vi "Big_LED_control.vi"() -> ()   [LabVIEW 2018]
uses:
  <instrlib>/niDCPower/nidcpower.llb/niDCPower Source Mode.ctl
  <instrlib>/niDCPower/nidcpower.llb/niDCPower Output Function.ctl
  AT lib/AmateurStepperMotor.dll
  <instrlib>/niDMM/nidmm.llb/niDMM Function.ctl
  <instrlib>/niDMM/nidmm.llb/niDMM Resolution in Digits.ctl
  <vilib>/Instr/_visa.llb/VISA Configure Serial Port (Instr).vi
  <instrlib>/niDMM/nidmm.llb/niDMM Configure Measurement Digits.vi
panel:
  out "Voltage Char 2":dbl(graph)=0.2558511793613434
  in  "I (np)":bool
  in  "Tab Control 2":enum32{"Шаговик и офир", "Служебная область"}(tab)
  in  "milliseconds to wait":u32=1000
  in  "Go To":dbl
  out "Ophir 1 Char":dbl(graph)=0.02
  in  "DecelerationTime, s":dbl=0.3
  in  "AccelerationTime, s":dbl=0.3
  in  "HoldOn":bool
  in  "Ophir 1 units":string(combo)="1000" caption="Units"
  out "Ophir 1 Over Range":bool caption="Over Range"
  out "Ophir 1 Optical Power":dbl=0.02 caption="Power" format="%#_4g"
  out "Ophir 1 MAX":dbl=0.02 caption="MAX" format="%#_5g"
  in  "Ophir 1 Clear":bool caption="Clear"
  in  "StepMultiplicationFactor":dbl=50.0
  in  "StepDivisor":i32(ring)=8 items=["D1"=1, "D2"=2, "D4"=4, "D8"=8, "D16"=16, "D32"=32]
  in  "Speed":dbl=250.0
  in  "Погнали!":bool
  in  "Стоп GoTo":bool
  out "Готово":bool
  out "Position":dbl=9.995
  in  "Ophir 1 Info":u16(ring)=1 caption="Info" items=["Device : ; s/n:", "Head : ; s/n:"]
  in  "new pos":dbl
  in  "set pos":bool
  out "Device Response":string="*\n"
  in  "Ophir 1 usb channel":i16 caption="usb channel"
  out "Ophir 1 dup Visa Session":refnum<visa-resource-name>="USB0::0x0BD3::0x0777::NI-VISA-60003::RAW" caption="dup Visa Session"
  in  "Ophir 1 Baud Rate (3:9600)":i16(ring)=3 caption="Baud Rate (3:9600)" items=["300", "1200", "4800", "9600", "19200", "38400"]
  out "Ophir 1 Real Optical Power":dbl=2e-05 format="%.6e"
  in  "Ophir 1 GPIB Address (10)":string="10" caption="GPIB Address (10)"
  in  "Ophir 1 Port Number (default 2)":i16=1 caption="Port Number (default 2)" min=0 max=20
  in  "Ophir 1 Select Communication Protocol":u16(ring) caption="Select Communication Protocol" items=["USB", "RS232", "GPIB"]
  out "Ophir 1 error out":errorcluster caption="error out"
  in  "Ophir 1 error in (no error)":errorcluster caption="error in (no error)"
  in  "Ophir 1 Wait":u32=100 caption="Wait"
  out "IsOpen":bool
  out "Ophir 1 Initialization":bool=TRUE caption="Initialization"
  in  "Tab Control":T1(tab)
  in  "шаговик":refnum<visa-resource-name>="COM8"
  in  "POWER":bool
  in  "Стоп":bool
  in  "Resource Name":refnum<k15>="PXI1Slot2" caption="Источник питания"
  in  "Амперметр":refnum<k15>="PXI1Slot4" caption="NI DMM 1"
  in  "V_MB, V":dbl=6.0 caption="voltage level" min=0.0 max=6.0 format="%_6p"
  in  "curlim_V_MB, A":dbl=0.3 caption="current limit" format="%_6p"
  out "chart_0":dbl(graph)=-0.00013853853853977013 caption="Waveform Chart 5"
  in  "voltlim_I_LED, V":dbl=2.1 caption="current limit" min=0.01 format="%_6p"
  in  "I_LED, A":dbl=0.010000000000000004 caption="voltage level" format="%_6p"
  out "chart_1":dbl(graph)=-0.0002744397184121777 caption="Waveform Chart 5"
  out "Current Char":dbl(graph)=0.0055655837059021
  in  "Arduino":refnum<visa-resource-name>="COM16"
  in  "Сегменты":bool[](array[boolean])=[FALSE, FALSE, FALSE, FALSE, FALSE, FALSE, FALSE, FALSE, FALSE, FALSE, FALSE, FALSE, FALSE, FALSE, FALSE, FALSE, FALSE, FALSE]
  in  "Вольтметр":refnum<k15>="PXI1Slot5" caption="NI DMM 1"
  out "Voltage Char":dbl(graph)=0.2558511793613434
  in  "wave_lenght":string="600"
  in  "Промер":bool caption="Промер сегмента"
  in  "NI DMM 1 Voltage Range 4":string(combo)="-1" caption="Range"
  in  "NI DMM 1 units 4":string(combo)="1" caption="Units"
  out "Voltage":dbl=0.2558511793613434 format="%_6g"
  in  "NI DMM 1 Current Range 3":string(combo)="1" caption="Range"
  in  "NI DMM 1 units 3":string(combo)="1000" caption="Units"
  out "Current":dbl format="%_6g"
  out "voltmes_V_MB, V":dbl=-0.00013853853853977013 caption="measurement" format="%_6g"
  out "curmes_V_MB, A":dbl caption="measurement" format="%_6g"
  out "curmes_I_LED, A":dbl=9.117163901385412e-07 caption="measurement" format="%_6g"
  out "voltmes_I_LED, V":dbl caption="measurement" format="%_6g"
  out "Разряд":dbl
  out "+/-":bool
  out "Power off":bool
  in  "Command":string="Cathode"
  in  "Записать":bool
  out "measure output \nfile refnum":refnum<file>
  out "Voltage, V":dbl=0.2558511793613434 caption="Measurement" format="%.5f"
  out "Current, A":dbl=5.5655837059021e-06 caption="Measurement" format="%.5f"
  out "Тип индикатора":string="Cathode"
  out "chart_2":dbl(graph)=0.0007584113885058215
  in  "V_RES, V":dbl caption="voltage level" format="%_6p"
  out "curmes_V_RES, A":dbl caption="measurement" format="%_6g"
  in  "curlim_V_RES, A":dbl=0.1 caption="current limit" min=0.01 format="%_6p"
  in  "measure path":path=path "C:/Users/user/Desktop/МСП/LabVIEW/LED_CONTROL_big_LED_ophir_24.12.24_1/Logs"
  out "Enum":enum16{"Exit", "4", "Промер", "2", "1"}(ring)
  out "№ об-ца":dbl
  out "Темп-ра":dbl
  out "Сегмент":string="n"
  out "voltmes_V_RES, V":dbl=0.0007584113885058215 caption="measurement" format="%_6g"
  in  "current level range":dbl=0.001 format="%#.6p"
  in  "1 - до 10 мА\n0 - от  30 мА":bool
  in  "II (Lm)":bool
  in  "III (jk)":bool
  in  "IV (gh)":bool
  in  "I - IV":bool
  # "Шаговик"
  # "Офир"
  # "(в мм)"
  # "Шаговик"
  # "Офир"
  # "position - это значение абсолютное"
  # "*если нужен ток меньше 10мА -> служебная область"
  # "j"
  # "c"
  # "d"
  # "e"
  # "g"
  # "h"
  # "a"
  # "b"
  # "f"
  # "k"
  # "L"
  # "m"
  # "n"
  # "p"
  # "dp"
  # "all"
  # "V_MB 5 В\nогрничение 300 м\n\nV_LED 2,1 В\nограничение 200 м"
  # "единицы мА\nrange 1 А"
  # "1. каждый сегмент включаем по отдельности, резистором постраиваем ток до 10 мА\n2. напряжение V_LED при этом не меняется\n3. в такоом положении промеряем сегменты по отдельности\n4. для промера всего индикатора сразу подстраиваем напряжение при неизменном положении резисторов\n5. ток всех индикаторов = ток одного сегмента (10 мА) * число сегментов (15)\n6. добиваемся этого увеличением V_LED"
  # "единицы В\nrange AUTO"
  # "регклировка суммарного тока через индикатор"
  # "24.063\n\n     I          U\n20 мА  1.3 В\n20 мА  1.4 В\n 7 мА   1.15 В"
  # "24.064\n\n     I          U\n10 мА  2 В\n10 мА  2.15 В\n 7 мА   1.9 В"
  # "автоматизировать подбор напряжения по известному максимальному напряжению и току. ОС по току сегмента"
  # "Р1:  +25°C\nР2:  - 60°C\nР3:  +85°C"
  # "регулировать ток в зависимости от температуры.\nс ростом температуры растет ток.\nпид-регулятор??"
  # "0. ввести номер образца\n1. включить нужный сегмент\n2. ввести его в поле справа\n3. вести температуру в поле слева\n4. нажать кнопку \"промер сегмента\""
  # "\"опрашивать кнопки не чаще, чем раз в секунду. сейчас кликать можно чаще, они загорятся, но ничего не произойдет\""
  # "24.067"
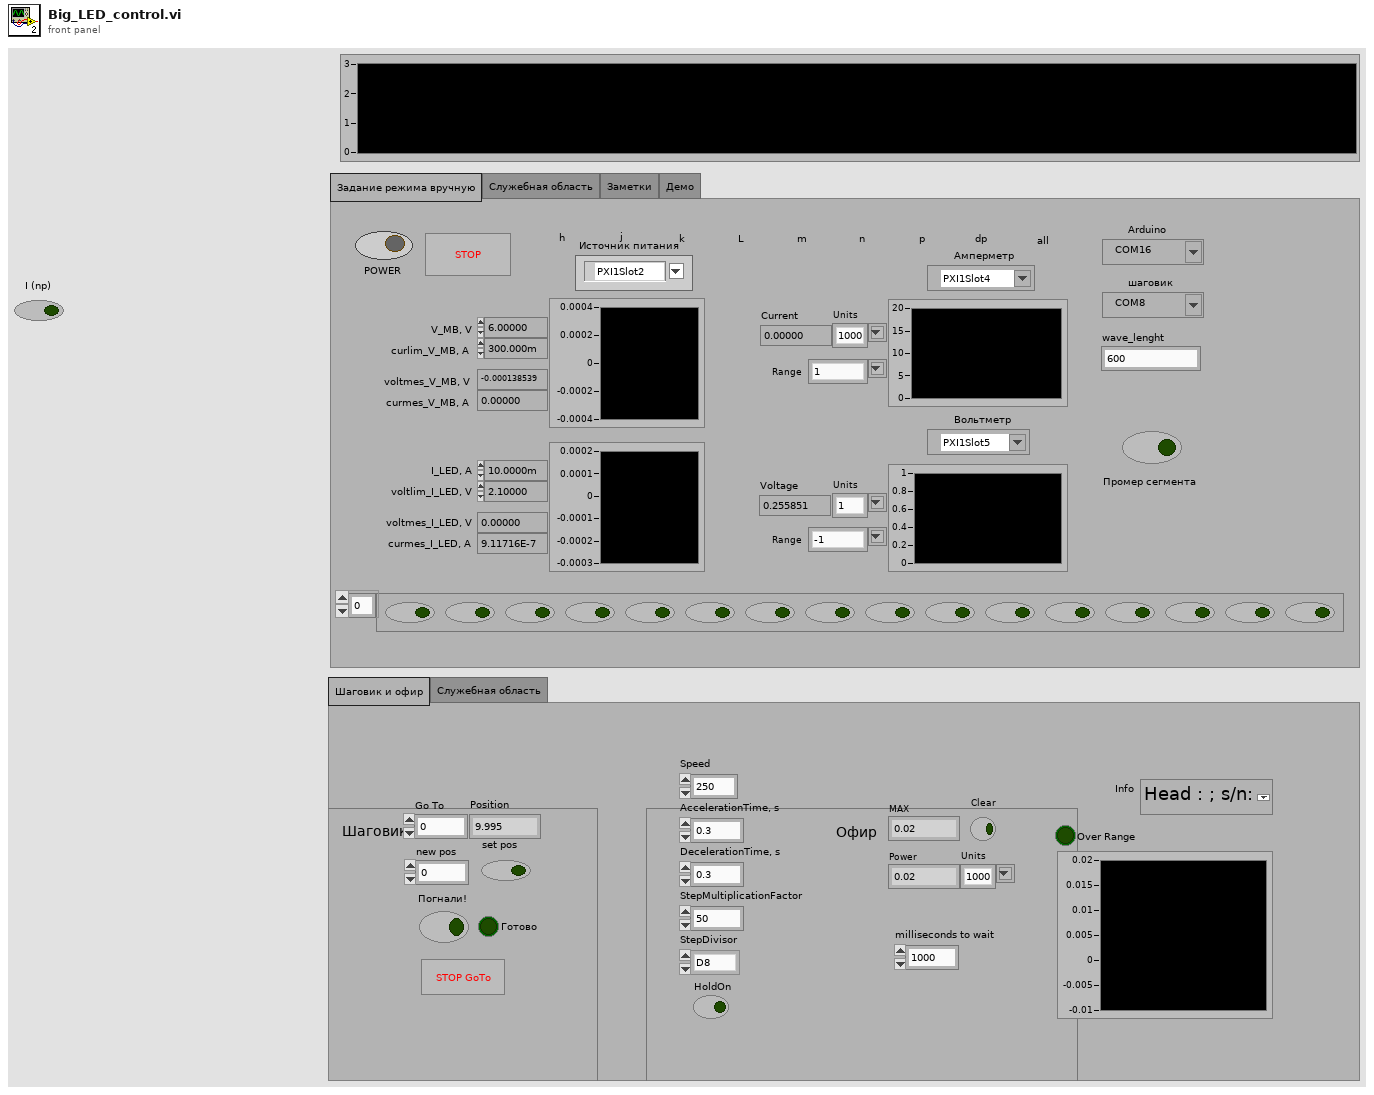
[diagram p1: front panel]
types:
  T1 = enum32{"Задание режима вручную", "Служебная область", "Заметки", "Демо"}
  T2 = enum16{"open", "replace", "create", "open or create", "replace or create", "replace or create with confirmation"}
  T3 = typedef "niDCPower Output Function.ctl" = i32
  T4 = typedef "niDCPower Source Mode.ctl" = i32
  T5 = typedef "niDMM Function.ctl" = enum16{"DC Volts", "AC Volts", "DC Current", "AC Current", "2-wire Resistance", "4-wire Resistance", "Diode", "Frequency", "Period", "AC Volts DC Coupled", "Capacitance", "Inductance", "Temperature"}
  T6 = typedef "niDMM Resolution in Digits.ctl" = dbl
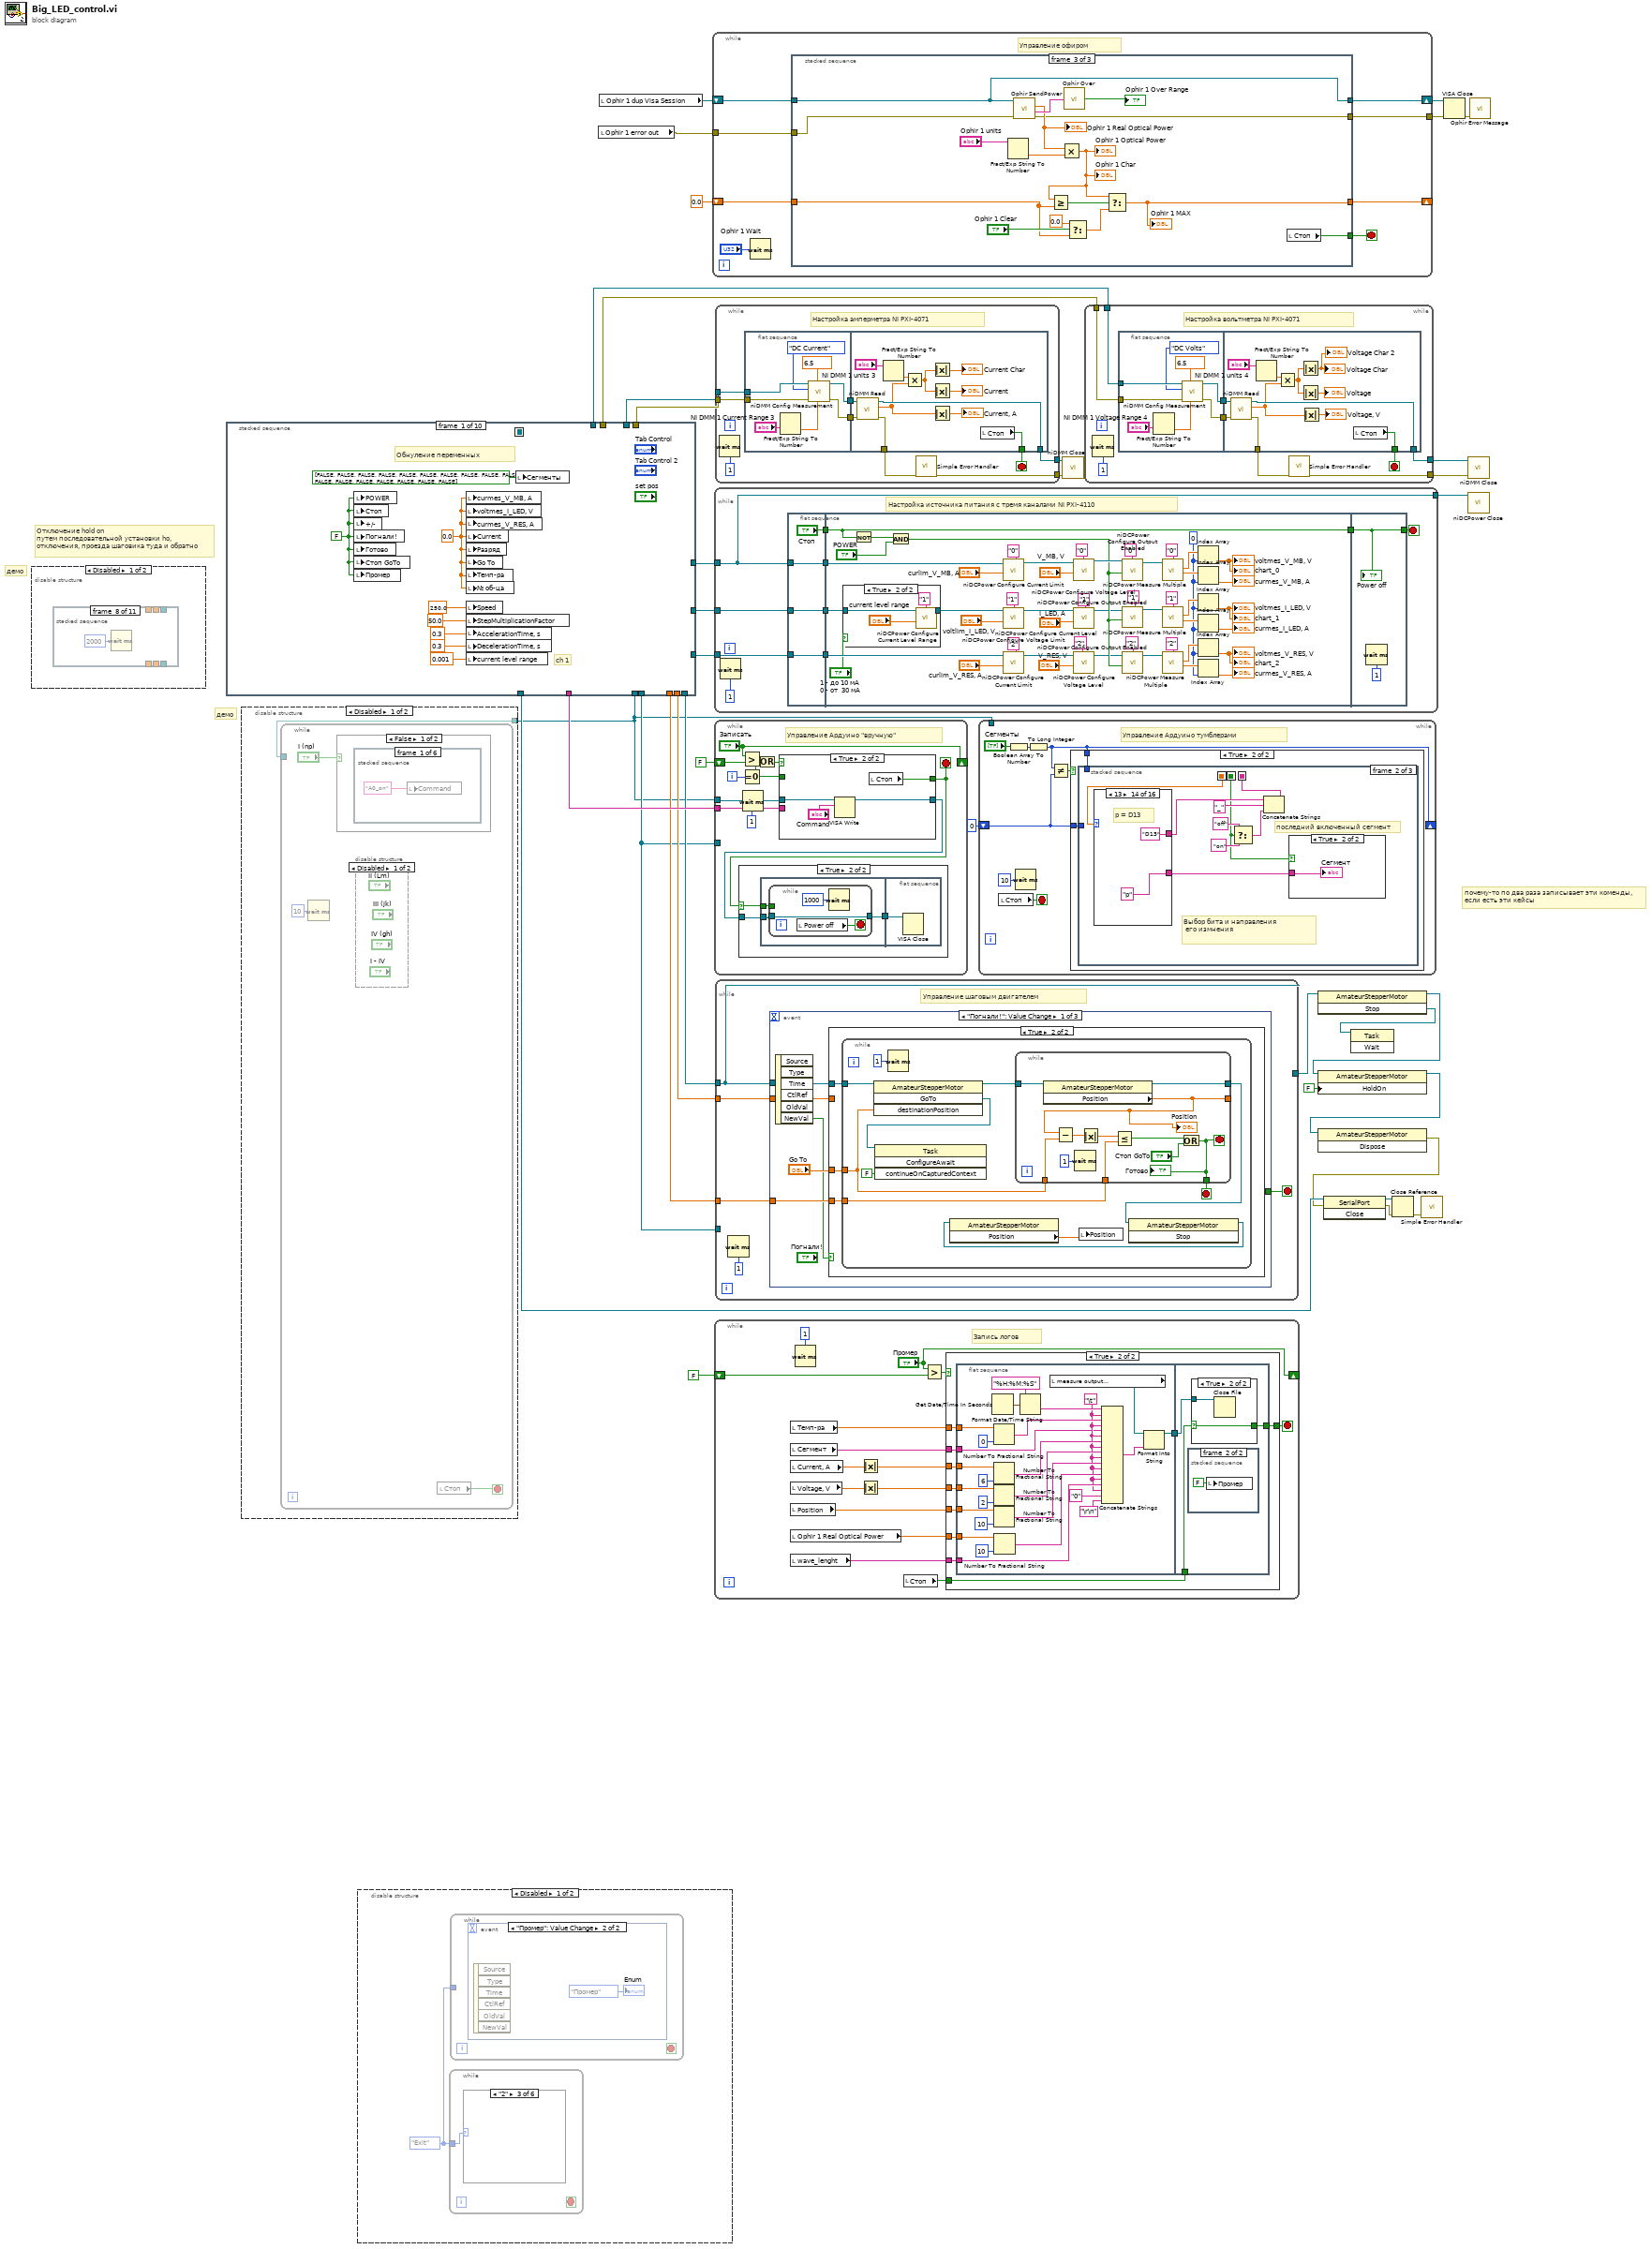
[diagram p0: block diagram]
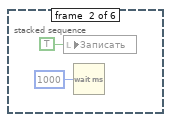
[diagram p3: hidden frame]
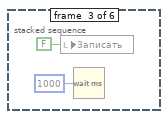
[diagram p4: hidden frame]
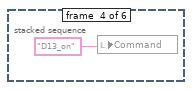
[diagram p5: hidden frame]
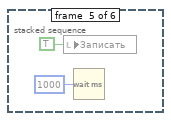
[diagram p6: hidden frame]
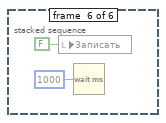
[diagram p7: hidden frame]
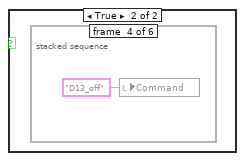
[diagram p8: hidden frame]
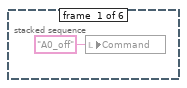
[diagram p9: hidden frame]
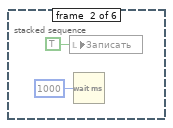
[diagram p10: hidden frame]
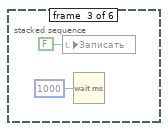
[diagram p11: hidden frame]
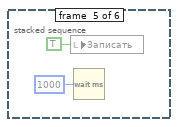
[diagram p12: hidden frame]
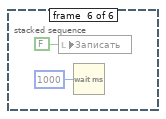
[diagram p13: hidden frame]
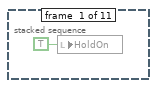
[diagram p15: hidden frame]
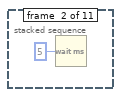
[diagram p16: hidden frame]
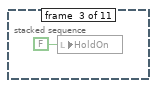
[diagram p17: hidden frame]
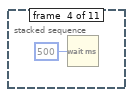
[diagram p18: hidden frame]
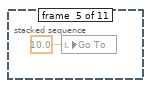
[diagram p19: hidden frame]
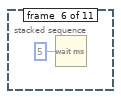
[diagram p20: hidden frame]
diagram:
  # "демо"
  # "демо"
  # "почему-то по два раза записывает эти коменды,\nесли есть эти кейсы"
  # "Отключение hold on\nпутем последовательной установки ho, \nотключения, проезда шаговика туда и обратно"
  n1 = disable-structure shown="Disabled" {
    frame Disabled {
      n2 = stacked-sequence {
        tunnel: _ -> [_ _ _ _ _ _ _ _ _ _ w50]
        tunnel: [_ _ _ _ _ _ _ _ _ _ w50] -> _
        tunnel: _ -> [_ _ _ _ _ _ _ _ _ _ w49]
        tunnel: [_ _ _ _ _ _ _ _ _ _ w49] -> _
        tunnel: [_ _ _ _ _ _ _ _ _ _ w48] -> _
        tunnel: _ -> [_ _ _ _ _ _ _ _ _ _ w48]
        frame #0 {
          n3 = local write "HoldOn"(TRUE ("HoldOn")) -> ()
        }
        frame #1 {
          n4 = Wait (ms)(milliseconds to wait=u32 5) -> ()  [unwired: 1 out]
        }
        frame #2 {
          n5 = local write "HoldOn"(FALSE ("HoldOn")) -> ()
        }
        frame #3 {
          n6 = Wait (ms)(milliseconds to wait=u32 500) -> ()  [unwired: 1 out]
        }
        frame #4 {
          n7 = local write "Go To"(10.0 ("Go To")) -> ()
        }
        frame #5 {
          n8 = Wait (ms)(milliseconds to wait=u32 5) -> ()  [unwired: 1 out]
        }
        frame #6 {
          n9 = local write "Погнали!"(TRUE ("Погнали!")) -> ()
        }
        frame #7 {
          n10 = Wait (ms)(milliseconds to wait=u32 2000) -> ()  [unwired: 1 out]
        }
        frame #8 {
          n11 = local write "Go To"(0.0 ("Go To")) -> ()
        }
        frame #9 {
          n12 = Wait (ms)(milliseconds to wait=u32 5) -> ()  [unwired: 1 out]
        }
        frame #10 {
          n13 = local write "Погнали!"(TRUE ("Погнали!")) -> ()
        }
      }
    }
    frame Enabled {
    }
  }
  n14 = stacked-sequence {
    seq-local: [_ _ _ _ _ _ w113 _ _ _] -> [_ _ _ _ _ _ _ w138 _ _]
    tunnel: [_ _ _ w68 _ _ _ _ _ _] -> w26
    tunnel: [_ w62 _ _ _ _ _ _ _ _] -> w37
    tunnel: [_ w61 _ _ _ _ _ _ _ _] -> w36
    tunnel: [_ _ _ _ w88 _ _ _ _ _] -> w1
    tunnel: [_ _ _ _ _ _ _ _ w144 _] -> w33
    tunnel: [_ _ w65 _ _ _ _ _ _ _] -> w32
    tunnel: [_ _ w64 _ _ _ _ _ _ _] -> w31
    tunnel: [_ _ _ _ _ _ _ w141 _ _] -> w3
    tunnel: [_ _ _ _ _ _ _ w139 _ _] -> w4
    tunnel: [_ _ _ _ _ _ _ w140 _ _] -> w5
    tunnel: [_ _ _ _ _ _ w115 _ _ _] -> w20
    tunnel: [_ _ _ w67 _ _ _ _ _ _] -> w8
    tunnel: [_ _ _ w66 _ _ _ _ _ _] -> w6
    tunnel: [_ _ _ _ _ _ _ _ _ w145] -> w2
    frame #0 {
      w52 = 0.0 ("currentmes_2")
      w53 = FALSE ("Стоп")
      # "ch 1"
      # "Обнуление переменных"
      n15 = local write "POWER"(w53) -> ()
      n16 = local write "Стоп"(w53) -> ()
      n17 = local write "+/-"(w53) -> ()
      n18 = local write "Погнали!"(w53) -> ()
      n19 = local write "Готово"(w53) -> ()
      n20 = local write "Стоп GoTo"(w53) -> ()
      n21 = local write "Промер"(w53) -> ()
      n22 = local write "curmes_V_MB, A"(w52) -> ()
      n23 = local write "voltmes_I_LED, V"(w52) -> ()
      n24 = local write "curmes_V_RES, A"(w52) -> ()
      n25 = local write "Current"(w52) -> ()
      n26 = local write "Разряд"(w52) -> ()
      n27 = local write "Go To"(w52) -> ()
      n28 = local write "Темп-ра"(w52) -> ()
      n29 = local write "№ об-ца"(w52) -> ()
      n30 = local write "Speed"(250.0 ("Speed")) -> ()
      n31 = local write "StepMultiplicationFactor"(50.0 ("StepMultiplicationFactor")) -> ()
      n32 = local write "AccelerationTime, s"(0.3 ("AccelerationTime, s")) -> ()
      n33 = local write "DecelerationTime, s"(0.3 ("DecelerationTime, s")) -> ()
      n34 = local write "current level range"(0.001 ("current level range")) -> ()
      n35 = local write "Сегменты"(bool[] [FALSE, FALSE, FALSE, FALSE, FALSE, FALSE, FALSE, FALSE, FALSE, FALSE, FALSE, FALSE, FALSE, FALSE, FALSE, FALSE, FALSE, FALSE] ("Сегменты")) -> ()
    }
    frame #1 {
      # "Инициализация амперметра"
      n36 = call <instrlib>:"niDMM Initialize.vi"("Instrument Descriptor"="Амперметр") -> ("error out"=w62:errorcluster, "instrument handle out"=w61:refnum<k15>)  [unwired: 9 in]
    }
    frame #2 {
      # "Инициализация вольтметра"
      n37 = call <instrlib>:"niDMM Initialize.vi"("Instrument Descriptor"="Вольтметр") -> ("error out"=w64:errorcluster, "instrument handle out"=w65:refnum<k15>)  [unwired: 9 in]
    }
    frame #3 {
      w73 = T3 1006 items=["DC Voltage"=1006, "DC Current"=1007, "Pulse Voltage"=1049, "Pulse Current"=1050] ("output function")
      w77 = T3 1007 items=["DC Voltage"=1006, "DC Current"=1007, "Pulse Voltage"=1049, "Pulse Current"=1050] ("output function")
      w78 = T3 1006 items=["DC Voltage"=1006, "DC Current"=1007, "Pulse Voltage"=1049, "Pulse Current"=1050] ("output function")
      w81 = T4 1020 items=["Single Point"=1020, "Sequence"=1021] ("source mode")
      # "Инициализация источника питания"
      n38 = call <instrlib>:"niDCPower Initialize.vi"("resource name"="Resource Name") -> ("instrument handle out"=w82:refnum<k15>)  [unwired: 3 in, 7 out]
      n39 = call <instrlib>:"niDCPower Configure Source Mode.vi"("source mode"=w81, "instrument handle"=w82) -> ("instrument handle out"=w72:refnum<k15>)  [unwired: 1 in, 8 out]
      n40 = call <instrlib>:"niDCPower Configure Output Function.vi"("output function"=w77, "channel name"="1", "instrument handle"=w72) -> ("instrument handle out"=w79:refnum<k15>)  [unwired: 7 in, 1 out]
      n41 = call <instrlib>:"niDCPower Configure Output Function.vi"("output function"=w73, "channel name"="2", "instrument handle"=w72) -> ("instrument handle out"=w74:refnum<k15>)  [unwired: 7 in, 1 out]
      n42 = call <instrlib>:"niDCPower Configure Output Function.vi"("output function"=w78, "channel name"="0", "instrument handle"=w72) -> ("instrument handle out"=w80:refnum<k15>)  [unwired: 7 in, 1 out]
      n43 = call <instrlib>:"niDCPower Configure Voltage Level.vi"("voltage level"=0.0, "channel name"="2", "instrument handle"=w74) -> ("instrument handle out"=w66:refnum<k15>)  [unwired: 7 in, 1 out]
      n44 = call <instrlib>:"niDCPower Configure Voltage Level.vi"("voltage level"=0.0, "channel name"="0", "instrument handle"=w80) -> ("instrument handle out"=w68:refnum<k15>)  [unwired: 7 in, 1 out]
      n45 = call <instrlib>:"niDCPower Configure Current Level.vi"("current level"=0.01, "channel name"="1", "instrument handle"=w79) -> ("instrument handle out"=w67:refnum<k15>)  [unwired: 7 in, 1 out]
    }
    frame #4 {
      # "Инициализация Ардуино"
      n46 = call-poly "VISA Configure Serial Port"("VISA resource name"="Arduino", "baud rate (9600)"=u32 9600) -> ("VISA resource name out"=w88:refnum<visa-resource-name>)  [unwired: 12 in, 1 out]
    }
    frame #5 {
      # "Инициализация офира"
      n47 = call "Ophir InitCom.vi"("GPIB Address (default 10)"="Ophir 1 GPIB Address (10)", "Communication (default USB 0)"="Ophir 1 Select Communication Protocol", "USB Channel number (default 0)"="Ophir 1 usb channel", "Port Number (default 2)"="Ophir 1 Port Number (default 2)", "error in (no error)"="Ophir 1 error in (no error)", "Baud Rate (3:9600)"="Ophir 1 Baud Rate (3:9600)") -> ("dup Visa Session"=w97:refnum<visa-resource-name>, "error out"=w96:errorcluster)  [unwired: 1 out]
      n48 = call "Ophir InstrInfo.vi"("Visa Session"=w97, "error in (no error)"=w96) -> ("dup Visa Session"=w109:refnum<visa-resource-name>, "Instrument Info"=w91:string, "error out"=w107:errorcluster)
      n49 = call "Ophir HeadInfo.vi"("Visa Session"=w109, "error in (no error)"=w107) -> ("error out"=w106:errorcluster, "dup Visa Session"=w108:refnum<visa-resource-name>, "Head Info"=w105:string)  [unwired: 6 out]
      n50 = call "Ophir InfoStrings.vi"("error in (no error)"=w106, "Head Info"=w105, "Instrument Info"=w91) -> ("error out"=w104:errorcluster, "Strings Array"=w103:string[])
      n51 = property on="Ophir 1 Info" class="Ring (strict)"("Strings []"=w103) -> ()  [unwired: 2 in, 2 out]
      n52 = call "Ophir ConfigDevice.vi"("Visa Session"=w108, "Measure Choice (0:Power)"=u16 0, "error in (no error)"=w104) -> ("dup Visa Session"=→"Ophir 1 dup Visa Session":refnum<visa-resource-name>, "OK ?"=→"Ophir 1 Initialization":bool, "error out"=→"Ophir 1 error out":errorcluster)  [unwired: 1 out]
    }
    frame #6 {
      w120 = 100 ("WriteTimeout")
      w124 = 1 items=["None", "One", "Two", "OnePointFive"] ("stopBits")
      w122 = 0 items=["None", "Odd", "Even", "Mark", "Space"] ("parity")
      # "убрали открытие порта. шаговик его и так сам откроет"
      # "Инициализация шаговика ч.1"
      n53 = constructor class="SerialPort"("portName"="шаговик", "baudRate"=57600, "parity"=w122, "dataBits"=8, "stopBits"=w124) -> (reference out=w119:refnum<k24>, error out=w118:errorcluster)  [unwired: 3 in, 6 out]
      n54 = property class="SerialPort"(reference=w119, error in=w118, "WriteTimeout"=w120, "ReadTimeout"=w120) -> (reference out=w115:refnum<k24>)  [unwired: 1 out]
      n55 = flat-sequence {
        tunnel: w115 -> [w131]
        tunnel: w114 -> [_]
        frame #0 {
          n56 = property class="SerialPort"(reference=w131) -> ("IsOpen"=→"IsOpen":bool)  [unwired: 1 in, 2 out]
        }
      }
      n57 = constructor class="AmateurStepperMotor"("serialPort"=w115) -> (reference out=w112:refnum<k24>, error out=w111:errorcluster)  [unwired: 3 in, 2 out]
      n58 = Not A Number/Path/Refnum?(number/path/refnum=w112) -> (NaN/Path/Refnum?=w116:bool)
      n59 = case shown="False" w116 {
        tunnel: w115 -> [_ w129]
        tunnel: [w125 w128] -> w114
        tunnel: [w126 w127] -> w113
        tunnel: w112 -> [w126 _]
        tunnel: w111 -> [w125 _]
        frame False {
        }
        frame True {
          n60 = constructor class="AmateurStepperMotor"("serialPort"=w129) -> (reference out=w127:refnum<k24>, error out=w128:errorcluster)  [unwired: 3 in, 2 out]
        }
      }
    }
    frame #7 {
      # "стоит допустить изменение\nтих параметров в цикле, а не только \nпри инициализации"
      # "это те самые 50 шагов за мм"
      # "Инициализация шаговика ч.2"
      n61 = property class="AmateurStepperMotor"(reference=w138, "Speed"="Speed", "StepDivisor"="StepDivisor", "StepMultiplicationFactor"="StepMultiplicationFactor", "AccelerationTime"="AccelerationTime, s", "DecelerationTime"="DecelerationTime, s", "HoldOn"="HoldOn") -> (reference out=w141:refnum<k24>, "Position"=w139:dbl, "PositioningPrecision"=w140:dbl)  [unwired: 1 in, 1 out]
    }
    frame #8 {
      # "Begin VI: ОК или ОА?"
      n62 = call "Begin.vi"() -> ("Темп-ра"=→"Темп-ра":dbl, "№ об-ца"=→"№ об-ца":dbl, "String"=w144:string)  [unwired: 6 in]
      "Тип индикатора" <- w144
      n63 = local write "Command"(w144) -> ()
    }
    frame #9 {
      w155 = "\t"
      # "Инициализация логов"
      n64 = local read "№ об-ца"() -> (w159:dbl)
      n65 = Number To Fractional String(number=w159, precision (6)=i16 0) -> (F-format string=w160:string)  [unwired: 2 in]
      n66 = Get Date/Time In Seconds() -> (seconds since 1Jan1904=w170:timestamp)
      n67 = Build Path(base path="measure path", name or relative path=w160) -> (appended path=w166:path)
      n68 = call <vilib>:"Check if File or Folder Exists.vi"("path"=w166) -> ("file or folder exists?"=w167:bool, "dup path"=w168:path)  [unwired: 8 in, 1 out]
      n69 = Format Date/Time String(time format string (%c)="MES %d. %m. %y %H.%M.%S", seconds (now)=w170) -> (date/time string=w171:string)  [unwired: 1 in]
      n70 = case shown="True" w167 {
        tunnel: w168 -> [w177 w178]
        tunnel: [w176 w178] -> w169
        frame False {
          n71 = Create Folder(path (use dialog)=w177) -> (created path=w176:path)  [unwired: 2 in, 2 out]
        }
        frame True {
        }
      }
      n72 = Concatenate Strings(w171, ".xls" ("string")) -> (w172:string)
      n73 = Build Path(base path=w169, name or relative path=w172) -> (appended path=w173:path)
      n74 = Open/Create/Replace File(file path (use dialog)=w173, operation (0:open)=T2."open or create", access (0:read/write)=enum16{"read/write", "read-only", "write-only"}."read/write") -> (refnum out=w174:refnum<file>)  [unwired: 3 in, 2 out]
      n75 = Set File Position(refnum=w174, from (0:start)=enum16{"start", "end", "current"}."end") -> (refnum out=w157:refnum<file>)  [unwired: 2 in, 1 out]
      n76 = Format Into String(initial string=w157, "Time" ("string"), w155, "Temperature, C" ("string"), w155, "Segment" ("string"), w155, "Current, mA" ("string"), w155, "Voltage, V" ("input 7"), w155, "Distance, m" ("string"), w155, "Power, W " ("string"), w155, "Wavelenght, nm" ("input 17"), w155, "Candlepower, kd" ("string"), "\r\n") -> (resulting string=w145:refnum<file>)  [unwired: 2 in, 1 out]
      "measure output \nfile refnum" <- w145
    }
  }
  n77 = disable-structure shown="Disabled" {
    disable-tunnel: w1 -> [w179 _]
    frame Disabled {
      n78 = while {
        tunnel: w179 -> [_]
        stop <- w181 stop-if-true
        n79 = Wait (ms)(milliseconds to wait=u32 10 ("millisecond timer value")) -> ()  [unwired: 1 out]
        n80 = case shown="False" "I (np)" {
          frame False {
            n81 = stacked-sequence {
              frame #0 {
                n82 = local write "Command"("A0_on" ("Command")) -> ()
              }
              frame #1 {
                n83 = local write "Записать"(TRUE ("Записать")) -> ()
                n84 = Wait (ms)(milliseconds to wait=u32 1000) -> ()  [unwired: 1 out]
              }
              frame #2 {
                n85 = local write "Записать"(FALSE ("Записать")) -> ()
                n86 = Wait (ms)(milliseconds to wait=u32 1000) -> ()  [unwired: 1 out]
              }
              frame #3 {
                n87 = local write "Command"("D13_on" ("Command")) -> ()
              }
              frame #4 {
                n88 = local write "Записать"(TRUE ("Записать")) -> ()
                n89 = Wait (ms)(milliseconds to wait=u32 1000) -> ()  [unwired: 1 out]
              }
              frame #5 {
                n90 = local write "Записать"(FALSE ("Записать")) -> ()
                n91 = Wait (ms)(milliseconds to wait=u32 1000) -> ()  [unwired: 1 out]
              }
            }
          }
          frame True {
            n92 = stacked-sequence {
              frame #0 {
                n93 = local write "Command"("A0_off" ("Command")) -> ()
              }
              frame #1 {
                n94 = local write "Записать"(TRUE ("Записать")) -> ()
                n95 = Wait (ms)(milliseconds to wait=u32 1000) -> ()  [unwired: 1 out]
              }
              frame #2 {
                n96 = local write "Записать"(FALSE ("Записать")) -> ()
                n97 = Wait (ms)(milliseconds to wait=u32 1000) -> ()  [unwired: 1 out]
              }
              frame #3 {
                n98 = local write "Command"("D13_off" ("Command")) -> ()
              }
              frame #4 {
                n99 = local write "Записать"(TRUE ("Записать")) -> ()
                n100 = Wait (ms)(milliseconds to wait=u32 1000) -> ()  [unwired: 1 out]
              }
              frame #5 {
                n101 = local write "Записать"(FALSE ("Записать")) -> ()
                n102 = Wait (ms)(milliseconds to wait=u32 1000) -> ()  [unwired: 1 out]
              }
            }
          }
        }
        n103 = disable-structure shown="Disabled" {
          frame Disabled {
          }
          frame Enabled {
          }
        }
        n104 = local read "Стоп"() -> (w181:bool)
      }
    }
    frame Enabled {
    }
  }
  n105 = disable-structure shown="Disabled" {
    frame Disabled {
      w203 = enum16{"Exit", "4", "Промер", "2", "1"}."Exit"
      n106 = while {
        tunnel: w203 -> [w204]
        stop <- _ stop-if-true
        n107 = case shown="\"2\"" w204 {
          frame "Exit", Default {
          }
          frame "4" {
          }
          frame "2" {
          }
          frame "2" {
          }
          frame "1" {
          }
          frame "Промер" {
          }
        }
      }
      n108 = while {
        tunnel: w203 -> [_]
        stop <- _ stop-if-true
        n109 = event shown="[1] \"Промер\": Value Change" {
          selector: _ -> [_ _]
          dyn-events: _ -> [_ _]
          timeout: _ -> [_ _]
          event Timeout {
            n110 = event-data() -> ()  [unwired: 1 in, 3 out]
          }
          event "Промер": Value Change {
            n111 = event-data() -> ()  [unwired: 1 in, 6 out]
            "Enum" <- enum16{"Exit", "4", "Промер", "2", "1"}."Промер" ("Enum")
          }
        }
      }
    }
    frame Enabled {
    }
  }
  n112 = local read "Ophir 1 error out"() -> (w24:errorcluster)
  n113 = local read "Ophir 1 dup Visa Session"() -> (w25:refnum<visa-resource-name>)
  n114 = while {
    tunnel: w24 -> [w212]
    shift-right: [w208] -> _
    shift-left: 0.0 ("t") -> [w211]
    shift-right: [w209] -> w18
    shift-left: w25 -> [w213]
    tunnel: [w207] -> w17
    stop <- w206 stop-if-true
    # "Управление офиром"
    n115 = Wait (ms)(milliseconds to wait="Ophir 1 Wait") -> ()  [unwired: 1 out]
    n116 = stacked-sequence {
      tunnel: w213 -> [w217 _ w220]
      tunnel: w212 -> [w216 _ w222]
      tunnel: w211 -> [_ _ w223]
      tunnel: [_ _ w220] -> w209
      tunnel: [_ _ w224] -> w208
      tunnel: [_ _ w221] -> w207
      tunnel: [_ _ w219] -> w206
      frame #0 {
        n117 = call "light_setWaveLenght.vi"("error in (no error)"=w216, "Visa Session"=w217, "wave_lenght"="wave_lenght") -> ("Device Response"=→"Device Response":string)  [unwired: 6 in, 2 out]
      }
      frame #1 {
        n118 = Wait (ms)(milliseconds to wait="milliseconds to wait") -> ()  [unwired: 1 out]
      }
      frame #2 {
        n119 = Fract/Exp String To Number(string="Ophir 1 units") -> (number=w227:dbl)  [unwired: 3 in, 1 out]
        n120 = call "Ophir SendPower.vi"("Visa Session"=w220, "error in (no error)"=w222) -> ("Value Number"=w226:dbl, "Value String"=w233:string, "error out"=w221:errorcluster)  [unwired: 1 out]
        "Ophir 1 Real Optical Power" <- w226
        n121 = Multiply(x=w226, y=w227) -> (x*y=w230:dbl)
        "Ophir 1 Char" <- w230
        "Ophir 1 Optical Power" <- w230
        n122 = Greater Or Equal?(x=w230, y=w223) -> (x >= y?=w231:bool)
        n123 = call "Ophir Over.vi"("Value String"=w233) -> ("Overrange"=→"Ophir 1 Over Range":bool)
        n124 = Select(t=0.0, s="Ophir 1 Clear", f=w223) -> (s? t:f=w229:dbl)
        n125 = Select(t=w230, s=w231, f=w229) -> (s? t:f=w224:dbl)
        "Ophir 1 MAX" <- w224
        n126 = local read "Стоп"() -> (w219:bool)
      }
    }
  }
  n127 = while {
    tunnel: w26 -> [w241]
    tunnel: [w241] -> w34
    tunnel: w8 -> [w238]
    tunnel: w6 -> [w235]
    stop <- w237 stop-if-true
    # "Настройка источника питания с тремя каналами NI PXI-4110"
    n128 = Wait (ms)(milliseconds to wait=u32 1) -> ()  [unwired: 1 out]
    n129 = flat-sequence {
      tunnel: w241 -> [w248]
      tunnel: [w248] -> w243
      tunnel: ["Стоп"] -> w242
      tunnel: [w246] -> w239
      tunnel: w238 -> [w246]
      tunnel: [w245] -> w236
      tunnel: w235 -> [w245]
      tunnel: w243 -> [w293]
      tunnel: w242 -> [w297]
      tunnel: [w297] -> w240
      tunnel: w239 -> [w261]
      tunnel: w236 -> [w256]
      tunnel: [w304] -> w237
      tunnel: w240 -> [w304]
      frame #0 {
      }
      frame #1 {
        w262 = 0 ("index")
        n130 = case shown="True" "1 - до 10 мА\n0 - от  30 мА" {
          tunnel: w261 -> [w298 w302]
          tunnel: [w298 w301] -> w260
          frame False {
          }
          frame True {
            n131 = call <instrlib>:"niDCPower Configure Current Level Range.vi"("current level range"="current level range", "channel name"="1", "instrument handle"=w302) -> ("instrument handle out"=w301:refnum<k15>)  [unwired: 7 in, 1 out]
          }
        }
        n132 = Not(x=w297) -> (.not. x?=w296:bool)
        n133 = And(x=w296, y="POWER") -> (x .and. y?=w292:bool)
        n134 = call <instrlib>:"niDCPower Configure Current Limit.vi"("current limit"="curlim_V_MB, A", "channel name"="0", "instrument handle"=w293) -> ("instrument handle out"=w283:refnum<k15>)  [unwired: 7 in, 1 out]
        n135 = call <instrlib>:"niDCPower Configure Voltage Limit.vi"("voltage limit"="voltlim_I_LED, V", "channel name"="1", "instrument handle"=w260) -> ("instrument handle out"=w287:refnum<k15>)  [unwired: 7 in, 1 out]
        n136 = call <instrlib>:"niDCPower Configure Current Limit.vi"("current limit"="curlim_V_RES, A", "channel name"="2", "instrument handle"=w256) -> ("instrument handle out"=w277:refnum<k15>)  [unwired: 7 in, 1 out]
        n137 = call <instrlib>:"niDCPower Configure Voltage Level.vi"("voltage level"="V_MB, V", "channel name"="0", "instrument handle"=w283) -> ("instrument handle out"=w294:refnum<k15>)  [unwired: 7 in, 1 out]
        n138 = call <instrlib>:"niDCPower Configure Current Level.vi"("current level"="I_LED, A", "channel name"="1", "instrument handle"=w287) -> ("instrument handle out"=w288:refnum<k15>)  [unwired: 7 in, 1 out]
        n139 = call <instrlib>:"niDCPower Configure Voltage Level.vi"("voltage level"="V_RES, V", "channel name"="2", "instrument handle"=w277) -> ("instrument handle out"=w278:refnum<k15>)  [unwired: 7 in, 1 out]
        n140 = call <instrlib>:"niDCPower Configure Output Enabled.vi"("output enabled"=w292, "channel name"="0", "instrument handle"=w294) -> ("instrument handle out"=w271:refnum<k15>)  [unwired: 7 in, 1 out]
        n141 = call <instrlib>:"niDCPower Configure Output Enabled.vi"("output enabled"=w292, "channel name"="1", "instrument handle"=w288) -> ("instrument handle out"=w264:refnum<k15>)  [unwired: 7 in, 1 out]
        n142 = call <instrlib>:"niDCPower Configure Output Enabled.vi"("output enabled"=w292, "channel name"="2", "instrument handle"=w278) -> ("instrument handle out"=w263:refnum<k15>)  [unwired: 7 in, 1 out]
        n143 = call <instrlib>:"niDCPower Measure Multiple.vi"("channel name"="0", "instrument handle"=w271) -> ("current measurements"=w269:dbl[], "voltage measurements"=w270:dbl[])  [unwired: 6 in, 2 out]
        n144 = call <instrlib>:"niDCPower Measure Multiple.vi"("channel name"="1", "instrument handle"=w264) -> ("current measurements"=w267:dbl[], "voltage measurements"=w268:dbl[])  [unwired: 6 in, 2 out]
        n145 = call <instrlib>:"niDCPower Measure Multiple.vi"("channel name"="2", "instrument handle"=w263) -> ("current measurements"=w265:dbl[], "voltage measurements"=w266:dbl[])  [unwired: 6 in, 2 out]
        n146 = Index Array(array=w270, index=w262) -> (element=→"chart_0" →"voltmes_V_MB, V":dbl)
        n147 = Index Array(array=w269, index=w262) -> (element=→"curmes_V_MB, A":dbl)
        n148 = Index Array(array=w268, index=w262) -> (element=→"chart_1" →"voltmes_I_LED, V":dbl)
        n149 = Index Array(array=w267, index=w262) -> (element=→"curmes_I_LED, A":dbl)
        n150 = Index Array(array=w266, index=w262) -> (element=→"chart_2" →"voltmes_V_RES, V":dbl)
        n151 = Index Array(array=w265, index=w262) -> (element=→"curmes_V_RES, A":dbl)
      }
      frame #2 {
        n152 = Wait (ms)(milliseconds to wait=u32 1) -> ()  [unwired: 1 out]
        "Power off" <- w304
      }
    }
  }
  n153 = while {
    tunnel: w1 -> [w312]
    shift-right: ["Записать"] -> _
    shift-left: FALSE ("Записать") -> [w314]
    tunnel: w33 -> [w310]
    tunnel: w2 -> [_]
    i -> [w311]
    stop <- w305 stop-if-true
    # "Управление Ардуино \"вручную\""
    n154 = Greater?(x="Записать", y=w314) -> (0:w308:bool)
    n155 = Equal To 0?(x=w311) -> (x = 0?=w307:bool)
    n156 = Wait (ms)(milliseconds to wait=u32 1) -> ()  [unwired: 1 out]
    n157 = Or(x=w308, y=w307) -> (x .or. y?=w309:bool)
    n158 = case shown="True" w309 {
      tunnel: w312 -> [w326 w331]
      tunnel: [w327 w330] -> w305
      tunnel: w310 -> [_ _]
      tunnel: w307 -> [_ _]
      tunnel: [w326 w328] -> w306
      frame False {
        n159 = local read "Стоп"() -> (w327:bool)
      }
      frame True {
        n160 = VISA Write(VISA resource name=w331, write buffer="Command") -> (VISA resource name out=w328:refnum<visa-resource-name>)  [unwired: 1 in, 2 out]
        n161 = local read "Стоп"() -> (w330:bool)
      }
    }
    n162 = case shown="True" w305 {
      selector: w305 -> [_ w316]
      tunnel: w306 -> [_ w318]
      frame False {
      }
      frame True {
        n163 = flat-sequence {
          tunnel: w318 -> [w321]
          tunnel: [w320] -> w317
          tunnel: w316 -> [w319]
          tunnel: w317 -> [w325]
          frame #0 {
            n164 = while {
              tunnel: w321 -> [w324]
              tunnel: [w324] -> w320
              tunnel: w319 -> [_]
              stop <- w322 stop-if-true
              n165 = local read "Power off"() -> (w322:bool)
              n166 = Wait (ms)(milliseconds to wait=u32 1000) -> ()  [unwired: 1 out]
            }
          }
          frame #1 {
            n167 = VISA Close(VISA resource name=w325) -> ()  [unwired: 1 in, 1 out]
          }
        }
      }
    }
  }
  n168 = while {
    shift-right: ["Промер"] -> _
    shift-left: FALSE ("Промер сегмента") -> [w344]
    stop <- w341 stop-if-true
    # "Запиcь логов"
    n169 = local read "Темп-ра"() -> (w337:dbl)
    n170 = local read "Сегмент"() -> (w338:string)
    n171 = local read "Current, A"() -> (w340:dbl)
    n172 = local read "Voltage, V"() -> (w339:dbl)
    n173 = local read "Position"() -> (w336:dbl)
    n174 = local read "Ophir 1 Real Optical Power"() -> (w334:dbl)
    n175 = local read "wave_lenght"() -> (w335:string)
    n176 = Wait (ms)(milliseconds to wait=u32 1) -> ()  [unwired: 1 out]
    n177 = Absolute Value(x=w340) -> (abs(x)=w332:dbl)
    n178 = Absolute Value(x=w339) -> (abs(x)=w333:dbl)
    n179 = local read "Стоп"() -> (w342:bool)
    n180 = Greater?(x="Промер", y=w344) -> (0:w345:bool)
    n181 = case shown="True" w345 {
      tunnel: w332 -> [_ w357]
      tunnel: w333 -> [_ w356]
      tunnel: w336 -> [_ w353]
      tunnel: w334 -> [_ w354]
      tunnel: w335 -> [_ w355]
      tunnel: w342 -> [w347 w351]
      tunnel: w337 -> [_ w350]
      tunnel: w338 -> [_ w349]
      tunnel: [w347 w348] -> w341
      frame False {
      }
      frame True {
        n182 = flat-sequence {
          tunnel: w357 -> [w375]
          tunnel: w356 -> [w374]
          tunnel: w355 -> [w372]
          tunnel: w354 -> [w371]
          tunnel: w353 -> [w370]
          tunnel: [w365] -> w352
          tunnel: w350 -> [w364]
          tunnel: w349 -> [w358]
          tunnel: w352 -> [w386]
          tunnel: w351 -> [w385]
          tunnel: [w384] -> w348
          frame #0 {
            w360 = "\t"
            n183 = Get Date/Time In Seconds() -> (seconds since 1Jan1904=w383:timestamp)
            n184 = Number To Fractional String(number=w364, precision (6)=i16 0) -> (F-format string=w362:string)  [unwired: 2 in]
            n185 = Number To Fractional String(number=w375, precision (6)=i16 6) -> (F-format string=w378:string)  [unwired: 2 in]
            n186 = Number To Fractional String(number=w374, precision (6)=i16 2) -> (F-format string=w377:string)  [unwired: 2 in]
            n187 = Number To Fractional String(number=w370, precision (6)=i16 10) -> (F-format string=w376:string)  [unwired: 2 in]
            n188 = Number To Fractional String(number=w371, precision (6)=i16 10) -> (F-format string=w373:string)  [unwired: 2 in]
            n189 = Format Date/Time String(time format string (%c)="%H:%M:%S", seconds (now)=w383) -> (date/time string=w381:string)  [unwired: 1 in]
            n190 = local read "measure output \nfile refnum"() -> (w379:refnum<file>)
            n191 = Concatenate Strings(w381, w360, w362, w360, w358, w360, w378, w360, w377, w360, w376, w360, w373, w360, w372, w360, "0" ("string"), "\r\n") -> (w380:string)
            n192 = Format Into String(initial string=w379, w380) -> (resulting string=w365:refnum<file>)  [unwired: 2 in, 1 out]
          }
          frame #1 {
            n193 = stacked-sequence {
              frame #0 {
                n194 = Wait (ms)(milliseconds to wait=u32 250) -> ()  [unwired: 1 out]
              }
              frame #1 {
                n195 = local write "Промер"(FALSE ("Промер")) -> ()
              }
            }
            n196 = case shown="True" w385 {
              selector: w385 -> [_ w390]
              tunnel: w386 -> [_ w391]
              tunnel: [FALSE w390] -> w384
              frame False {
              }
              frame True {
                n197 = Close File(refnum=w391) -> ()  [unwired: 1 in, 2 out]
              }
            }
          }
        }
      }
    }
  }
  n198 = while {
    tunnel: [w398] -> w27
    tunnel: w36 -> [w396]
    tunnel: w37 -> [w395]
    tunnel: [w392] -> w28
    stop <- w394 stop-if-true
    # "Настройка амперметра NI PXI-4071"
    n199 = Wait (ms)(milliseconds to wait=u32 1) -> ()  [unwired: 1 out]
    n200 = flat-sequence {
      tunnel: [w405] -> w400
      tunnel: w396 -> [w403]
      tunnel: w395 -> [w407]
      tunnel: [w404] -> w399
      tunnel: w400 -> [w417]
      tunnel: w399 -> [w420]
      tunnel: [w416] -> w394
      tunnel: [w415] -> w392
      tunnel: [w414] -> w393
      frame #0 {
        w401 = T6 6.5 items=["3 1/2"=3.5, "4 1/2"=4.5, "5 1/2"=5.5, "6 1/2"=6.5, "7 1/2"=7.5] ("Resolution in Digits")
        n201 = Fract/Exp String To Number(string="NI DMM 1 Current Range 3") -> (number=w406:dbl)  [unwired: 3 in, 1 out]
        n202 = call-poly <instrlib>:"niDMM Config Measurement.vi"("Range"=w406, "Resolution in Digits"=w401, "error in (no error)"=w407, "Function"=niDMM_Function."DC Current" ("Measurement Type"), "instrument handle"=w403) -> ("error out"=w404:errorcluster, "instrument handle out"=w405:refnum<k15>)  [unwired: 5 in]
      }
      frame #1 {
        n203 = call <instrlib>:"niDMM Read.vi"("error in (no error)"=w420, "instrument handle"=w417) -> ("error out"=w414:errorcluster, "Measurement"=w409:dbl, "instrument handle out"=w415:refnum<k15>)  [unwired: 7 in]
        n204 = Fract/Exp String To Number(string="NI DMM 1 units 3") -> (number=w418:dbl)  [unwired: 3 in, 1 out]
        n205 = Multiply(x=w418, y=w409) -> (x*y=w411:dbl)
        n206 = Absolute Value(x=w411) -> (abs(x)=→"Current Char":dbl)
        n207 = Absolute Value(x=w411) -> (abs(x)=→"Current":dbl)
        n208 = Absolute Value(x=w409) -> (abs(x)=→"Current, A":dbl)
        n209 = local read "Стоп"() -> (w416:bool)
      }
    }
    n210 = call <vilib>:"Simple Error Handler.vi"("error in (no error)"=w393) -> ("error out"=w398:errorcluster)  [unwired: 1 in, 7 out]
  }
  n211 = while {
    tunnel: w3 -> [w422]
    tunnel: w5 -> [w424]
    tunnel: [w422] -> w7
    tunnel: w4 -> [w425]
    tunnel: w2 -> [_]
    stop <- w421 stop-if-true
    # "Управление шаговым двигателем"
    n212 = Wait (ms)(milliseconds to wait=u32 1) -> ()  [unwired: 1 out]
    n213 = event shown="[0] \"Погнали!\": Value Change" {
      selector: _ -> [_ _ _]
      dyn-events: _ -> [_ _ _]
      timeout: _ -> [_ _ _]
      tunnel: w422 -> [w430 w458 _]
      tunnel: w425 -> [w429 _ _]
      tunnel: w424 -> [w428 _ _]
      tunnel: [_ _ w464] -> w421
      event "Погнали!": Value Change {
        n214 = event-data() -> ("NewVal"=w426:bool)  [unwired: 1 in, 5 out]
        n215 = case shown="True" w426 {
          tunnel: "Go To" -> [_ w434]
          tunnel: w430 -> [_ w433]
          tunnel: w429 -> [_ _]
          tunnel: w428 -> [_ w432]
          frame False {
            n216 = Wait (ms)(milliseconds to wait=u32 1) -> ()  [unwired: 1 out]
          }
          frame True {
            n217 = while {
              tunnel: w434 -> [w441]
              tunnel: w433 -> [w442]
              tunnel: w432 -> [w444]
              stop <- w445 stop-if-true
              n218 = invoke class="AmateurStepperMotor" method="GoTo"(reference=w442, "destinationPosition"=w441) -> (reference out=w437:refnum<k24>, "GoTo"=w440:refnum<k24>)  [unwired: 2 in, 2 out]
              n219 = invoke class="Task" method="ConfigureAwait"(reference=w440, "continueOnCapturedContext"=FALSE) -> ()  [unwired: 2 in, 4 out]
              n220 = Wait (ms)(milliseconds to wait=u32 1) -> ()  [unwired: 1 out]
              n221 = while {
                tunnel: [w446] -> _
                tunnel: [w448] -> w438
                tunnel: [w450] -> w445
                tunnel: w441 -> [w455]
                tunnel: w444 -> [w453]
                tunnel: w437 -> [w447]
                stop <- w450 stop-if-true
                n222 = property class="AmateurStepperMotor"(reference=w447) -> (reference out=w448:refnum<k24>, "Position"=w446:dbl)  [unwired: 1 in, 1 out]
                "Position" <- w446
                n223 = Subtract(x=w446, y=w455) -> (x-y=w456:dbl)
                n224 = Wait (ms)(milliseconds to wait=u32 1) -> ()  [unwired: 1 out]
                n225 = Absolute Value(x=w456) -> (abs(x)=w454:dbl)
                n226 = Less Or Equal?(x=w454, y=w453) -> (x <= y?=w452:bool)
                n227 = Or(x=w452, y="Стоп GoTo") -> (x .or. y?=w450:bool)
                "Готово" <- w450
              }
              n228 = invoke class="AmateurStepperMotor" method="Stop"(reference=w438) -> (reference out=w436:refnum<k24>)  [unwired: 2 in, 2 out]
              n229 = property class="AmateurStepperMotor"(reference=w436) -> ("Position"=w435:dbl)  [unwired: 1 in, 2 out]
              n230 = local write "Position"(w435) -> ()
            }
          }
        }
      }
      event "set pos": Value Change {
        n231 = event-data() -> ("NewVal"=w459:bool)  [unwired: 1 in, 5 out]
        n232 = case shown="False" w459 {
          tunnel: w458 -> [_ w463]
          tunnel: "new pos" -> [_ w462]
          frame False {
          }
          frame True {
            n233 = property class="AmateurStepperMotor"(reference=w463, "Position"=w462) -> (reference out=w461:refnum<k24>)  [unwired: 1 in, 1 out]
            n234 = property class="AmateurStepperMotor"(reference=w461) -> ("Position"=w460:dbl)  [unwired: 1 in, 2 out]
            n235 = local write "Position"(w460) -> ()
          }
        }
      }
      event "Стоп": Value Change {
        n236 = event-data() -> ()  [unwired: 1 in, 6 out]
        n237 = local read "Стоп"() -> (w464:bool)
      }
    }
  }
  n238 = while {
    shift-right: [w465] -> _
    shift-left: 0 -> [w467]
    tunnel: w1 -> [_]
    stop <- w471 stop-if-true
    # "Управление Ардуино тумблерами"
    n239 = local read "Стоп"() -> (w471:bool)
    n240 = Boolean Array To Number(Boolean array="Сегменты") -> (number=w466:u32)
    n241 = Wait (ms)(milliseconds to wait=u32 10 ("millisecond timer value")) -> ()  [unwired: 1 out]
    n242 = To Long Integer(number=w466) -> (32bit integer=w465:i32)
    n243 = Not Equal?(x=w465, y=w467) -> (x != y?=w469:bool)
    n244 = case shown="True" w469 {
      tunnel: w465 -> [_ w472]
      tunnel: w467 -> [_ w473]
      frame False {
      }
      frame True {
        n245 = stacked-sequence {
          seq-local: [w476 _ _] -> [_ w481 _]
          seq-local: [w474 _ _] -> [_ w485 _]
          seq-local: [_ w486 _] -> [_ _ w523]
          tunnel: w472 -> [w478 _ _]
          tunnel: w473 -> [w477 _ _]
          frame #0 {
            # "Детектирвоание позиции и\nнаправления изменения бита"
            n246 = Subtract(x=w478, y=w477) -> (x-y=w479:i32)
            n247 = To Double Precision Float(number=w479) -> (double precision float=w480:dbl)
            n248 = Greater Than 0?(x=w479) -> (x > 0?=w476:bool)
            "+/-" <- w476
            n249 = Absolute Value(x=w480) -> (abs(x)=w475:dbl)
            n250 = Logarithm Base 2(1:w475) -> (0:w474:dbl)
            "Разряд" <- w474
          }
          frame #1 {
            # "последний включенный сегмент"
            # "Выбор бита и направления\n его измнения"
            n251 = case shown="13" w485 {
              tunnel: ["D10" "D9" "D5" "D8" "D11" "D12" "A1" "D4" "A5" "A4" "A3" "A2" "A0" "D13" "D3" "All"] -> w483
              tunnel: ["a" "b" "c" "d" "e" "f" "g" "h" "j" "k" "L" "m" "n" "p" "dp" "All"] -> w482
              frame 0, Default {
                # "a = D10"
              }
              frame 1 {
                # "b = D9"
              }
              frame 2 {
                # "c = D5"
              }
              frame 3 {
                # "d = D8"
              }
              frame 4 {
                # "e = D11"
              }
              frame 5 {
                # "f = D12"
              }
              frame 6 {
                # "g = A1"
              }
              frame 7 {
                # "h = D4"
              }
              frame 8 {
                # "j = A5"
              }
              frame 9 {
                # "k = A4"
              }
              frame 10 {
                # "L = A3"
              }
              frame 11 {
                # "m = A2"
              }
              frame 12 {
                # "n = A0"
              }
              frame 13 {
                # "p = D13"
              }
              frame 14 {
                # "dp = D3"
              }
              frame 15 {
              }
            }
            n252 = Select(t="off", s=w481, f="on") -> (s? t:f=w484:string)
            n253 = Concatenate Strings(w483, "_" ("string"), w484) -> (w486:string)
            n254 = case shown="True" w481 {
              tunnel: w482 -> [_ w490]
              frame False {
              }
              frame True {
                "Сегмент" <- w490
              }
            }
          }
          frame #2 {
            # "Передача команды в Ардуино"
            n255 = disable-structure shown="Disabled" {
              disable-tunnel: w523 -> [w525 _]
              frame Disabled {
                n256 = Equal?(x=w525, y="All_off") -> (x = y?=w528:bool)
                n257 = Equal?(x=w525, y="All_on") -> (x = y?=w526:bool)
                n258 = case shown="True" w528 {
                  frame False {
                  }
                  frame True {
                    n259 = local write "Сегменты"(bool[] [TRUE, TRUE, TRUE, TRUE, TRUE, TRUE, TRUE, TRUE, TRUE, TRUE, TRUE, TRUE, TRUE, TRUE, TRUE, TRUE] ("Сегменты")) -> ()
                  }
                }
                n260 = case shown="True" w526 {
                  frame False {
                  }
                  frame True {
                    n261 = local write "Сегменты"(bool[] [FALSE, FALSE, FALSE, FALSE, FALSE, FALSE, FALSE, FALSE, FALSE, FALSE, FALSE, FALSE, FALSE, FALSE, FALSE, FALSE] ("Сегменты")) -> ()
                  }
                }
              }
              frame Enabled {
              }
            }
            n262 = stacked-sequence {
              tunnel: w523 -> [w531 _ _]
              frame #0 {
                n263 = local write "Command"(w531) -> ()
              }
              frame #1 {
                n264 = local write "Записать"(TRUE ("Записать")) -> ()
                n265 = Wait (ms)(milliseconds to wait=u32 1000) -> ()  [unwired: 1 out]
              }
              frame #2 {
                n266 = local write "Записать"(FALSE ("Записать")) -> ()
                n267 = Wait (ms)(milliseconds to wait=u32 1000) -> ()  [unwired: 1 out]
              }
            }
          }
        }
      }
    }
  }
  n268 = call <instrlib>:"niDMM Close.vi"("error in (no error)"=w27, "instrument handle"=w28) -> ()  [unwired: 9 in, 1 out]
  n269 = while {
    tunnel: [w542] -> w29
    tunnel: w32 -> [w540]
    tunnel: w31 -> [w539]
    tunnel: [w536] -> w30
    stop <- w538 stop-if-true
    # "Настройка вольтметра NI PXI-4071"
    n270 = Wait (ms)(milliseconds to wait=u32 1) -> ()  [unwired: 1 out]
    n271 = flat-sequence {
      tunnel: [w549] -> w544
      tunnel: w540 -> [w547]
      tunnel: w539 -> [w551]
      tunnel: [w548] -> w543
      tunnel: w544 -> [w561]
      tunnel: w543 -> [w564]
      tunnel: [w560] -> w538
      tunnel: [w559] -> w536
      tunnel: [w558] -> w537
      frame #0 {
        w545 = T6 6.5 items=["3 1/2"=3.5, "4 1/2"=4.5, "5 1/2"=5.5, "6 1/2"=6.5, "7 1/2"=7.5] ("Resolution in Digits")
        n272 = Fract/Exp String To Number(string="NI DMM 1 Voltage Range 4") -> (number=w550:dbl)  [unwired: 3 in, 1 out]
        n273 = call-poly <instrlib>:"niDMM Config Measurement.vi"("Range"=w550, "Resolution in Digits"=w545, "error in (no error)"=w551, "Function"=niDMM_Function."DC Volts" ("Measurement Type"), "instrument handle"=w547) -> ("error out"=w548:errorcluster, "instrument handle out"=w549:refnum<k15>)  [unwired: 5 in]
      }
      frame #1 {
        n274 = call <instrlib>:"niDMM Read.vi"("error in (no error)"=w564, "instrument handle"=w561) -> ("error out"=w558:errorcluster, "Measurement"=w554:dbl, "instrument handle out"=w559:refnum<k15>)  [unwired: 7 in]
        n275 = Fract/Exp String To Number(string="NI DMM 1 units 4") -> (number=w562:dbl)  [unwired: 3 in, 1 out]
        n276 = Multiply(x=w562, y=w554) -> (x*y=w556:dbl)
        n277 = Absolute Value(x=w556) -> (abs(x)=→"Voltage Char" →"Voltage Char 2":dbl)
        n278 = Absolute Value(x=w556) -> (abs(x)=→"Voltage":dbl)
        n279 = Absolute Value(x=w554) -> (abs(x)=→"Voltage, V":dbl)
        n280 = local read "Стоп"() -> (w560:bool)
      }
    }
    n281 = call <vilib>:"Simple Error Handler.vi"("error in (no error)"=w537) -> ("error out"=w542:errorcluster)  [unwired: 1 in, 7 out]
  }
  n282 = invoke class="AmateurStepperMotor" method="Stop"(reference=w7) -> (reference out=w14:refnum<k24>, "Stop"=w15:refnum<k24>)  [unwired: 2 in, 1 out]
  n283 = property class="AmateurStepperMotor"(reference=w14, "HoldOn"=FALSE) -> (reference out=w13:refnum<k24>)  [unwired: 1 in, 1 out]
  n284 = invoke class="AmateurStepperMotor" method="Dispose"(reference=w13) -> (error out=w10:errorcluster)  [unwired: 2 in, 2 out]
  n285 = invoke class="SerialPort" method="Close"(reference=w20, error in=w10) -> (reference out=w9:refnum<k24>, error out=w11:errorcluster)  [unwired: 1 in, 1 out]
  n286 = invoke class="Task" method="Wait"(reference=w15) -> ()  [unwired: 2 in, 3 out]
  n287 = Close Reference(reference=w9, error in (no error)=w11) -> (error out=w12:errorcluster)
  n288 = call <vilib>:"Simple Error Handler.vi"("error in (no error)"=w12) -> ()  [unwired: 1 in, 8 out]
  n289 = VISA Close(VISA resource name=w18, error in (no error)=w17) -> (error out=w22:errorcluster)
  n290 = call <instrlib>:"niDMM Close.vi"("error in (no error)"=w29, "instrument handle"=w30) -> ()  [unwired: 9 in, 1 out]
  n291 = call <instrlib>:"niDCPower Close.vi"("instrument handle"=w34) -> ()  [unwired: 10 in, 1 out]
  n292 = call "Ophir Error Message.vi"("error in (no error)"=w22) -> ()  [unwired: 3 in, 4 out]
